vi "Current_Setpt_DriDir_Handler.vi"(10 "Drive Direction":enum16{"Clockwise", "Counterclockwise"}(ring), 11 "Current Setpoint (Amps)":dbl) -> (3 "Numeric":i16)   [LabVIEW 2011]
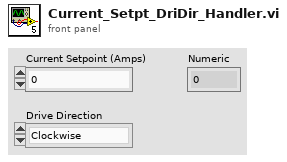
[diagram p1: front panel]
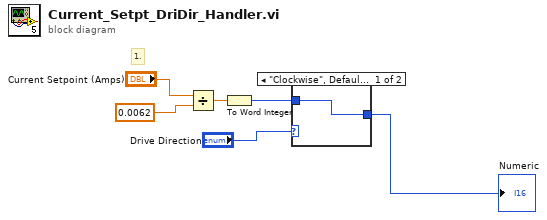
[diagram p0: block diagram]
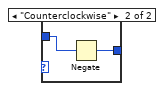
[diagram p2: hidden frame]
diagram:
  # "1."
  n1 = Divide(x="Current Setpoint (Amps)", y=0.0062) -> (x/y=w3:dbl)
  n2 = To Word Integer(number=w3) -> (16bit integer=w5:i16)
  n3 = case shown="\"Clockwise\", Default" "Drive Direction" {
    tunnel: w5 -> [w7 w9]
    tunnel: [w7 w8] -> w6
    frame "Clockwise", Default {
    }
    frame "Counterclockwise" {
      n4 = Negate(x=w9) -> (-x=w8:i16)
    }
  }
  "Numeric" <- w6
